vi "PresetSave.vi"(7 "Save time?":bool, 8 "error in (no error)":errorcluster, 9 "PresetFilePath":path, 10 "GViewer-Queue":refnum<queue>, 11 "Presets":T1[](array[typedef]) {"max" format="%#_3p"; "min" format="%#_3p"}) -> (0 "error out":errorcluster)   [LabVIEW 2020, in "Sgraph_lib_V1.lvlib" / "Gviewer.lvclass"]
doc: "Andre Koelewijn, 5 feb 2021\n\nPreset TAGs Preset"
uses:
  Gviewer.lvclass
  controls/EditTagOneTag.ctl
  controls/Typedef_Gserver-Replies.ctl
  controls/Typedef_ServerActions.ctl
  controls/Typedef_PresetSave.ctl
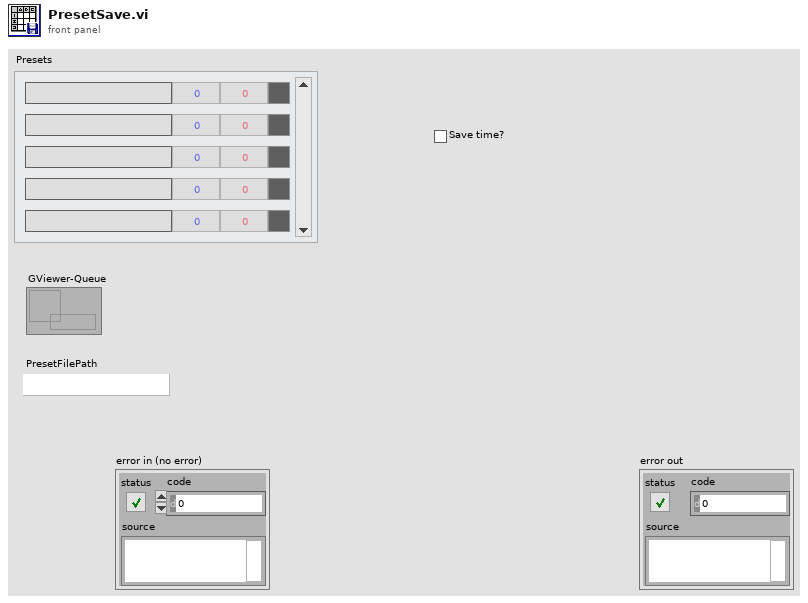
[diagram p1: front panel]
types:
  T1 = typedef "Sgraph_lib_V1.lvlib/Gviewer.lvclass/EditTagOneTag.ctl" = cluster{"TAG":string, "min":dbl, "max":dbl, "Color":u32}
  T2 = typedef "Sgraph_lib_V1.lvlib/Gviewer.lvclass/Typedef_PresetSave.ctl" = cluster{"Save time?":bool, "Presets":T1[], "PresetFilePath":path}
  T3 = typedef "Sgraph_lib_V1.lvlib/Gviewer.lvclass/Typedef_ServerActions.ctl" = enum16{"GraphUpdate", "SendAllTags", "SendIniPath", "SetGeneralOptions", "EditTagsOpen", "EditTagsPresetSave", "EditTagsPresetLoad", "EditTagsClose", "NewTagSelection", "AutoScale", "DBeditStatus", "DBsaveConfirm", "ExitGraph"}
  T4 = typedef "Typedef_Gserver-Replies.ctl" = cluster{"ServerActions":T3, "data":variant, "Source":string, "Time Stamp":timestamp}
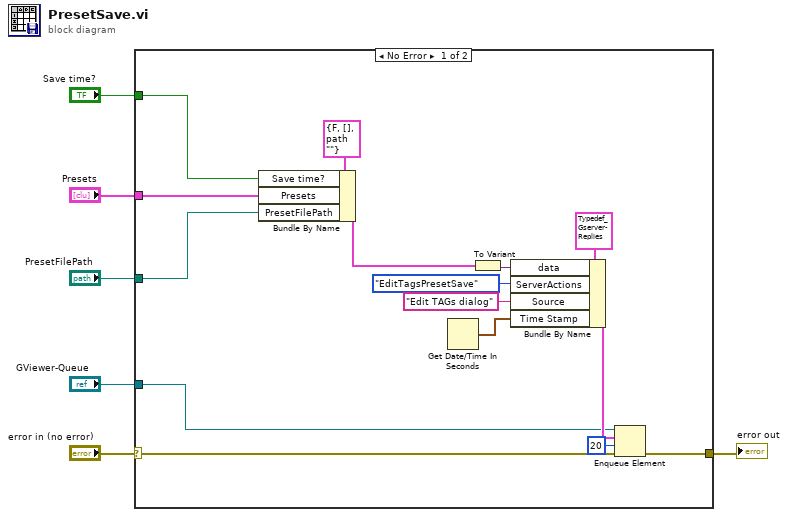
[diagram p0: block diagram]
diagram:
  n1 = case shown="No Error" "error in (no error)" {
    selector: "error in (no error)" -> [w16 w22]
    tunnel: [w15 w22] -> w5
    tunnel: "Save time?" -> [w13 _]
    tunnel: "Presets" -> [w12 _]
    tunnel: "PresetFilePath" -> [w11 _]
    tunnel: "GViewer-Queue" -> [w10 _]
    frame No Error {
      n2 = Bundle By Name(cluster=T2 {"Save time?"=FALSE, "Presets"=[], "PresetFilePath"=path ""} ("PresetSave"), "Save time?"=w13, "Presets"=w12, "PresetFilePath"=w11) -> (w7:T2)
      n3 = Get Date/Time In Seconds() -> (seconds since 1Jan1904=w21:timestamp)
      n4 = To Variant(anything=w7) -> (Variant=w8:variant)
      n5 = Bundle By Name(cluster=T4 {"ServerActions"=enum."GraphUpdate", "data"=variant, "Source"="", "Time Stamp"=timestamp(0 s since 1904-01-01)} ("element"), "data"=w8, "ServerActions"=Typedef_ServerActions."EditTagsPresetSave", "Source"="Edit TAGs dialog", "Time Stamp"=w21) -> (w20:T4)
      n6 = Enqueue Element(queue=w10, element=w20, timeout in ms (-1)=20, error in (no error)=w16) -> (error out=w15:errorcluster)  [unwired: 2 out]
    }
    frame Error {
    }
  }
  "error out" <- w5
